vi "CRYEmpty Listbox.vi"   [LabVIEW 2013]
uses:
  Global/CRYCurve Library Global.vi
panel:
  # "Empty Curve Library Listbox"
types:
  T1 = cluster{"Left Cell String":string, "Child Text":string[], "Child Tag":string, "Item Indent":i32, "Child Only?":bool, "Glyph Index":i32}[]
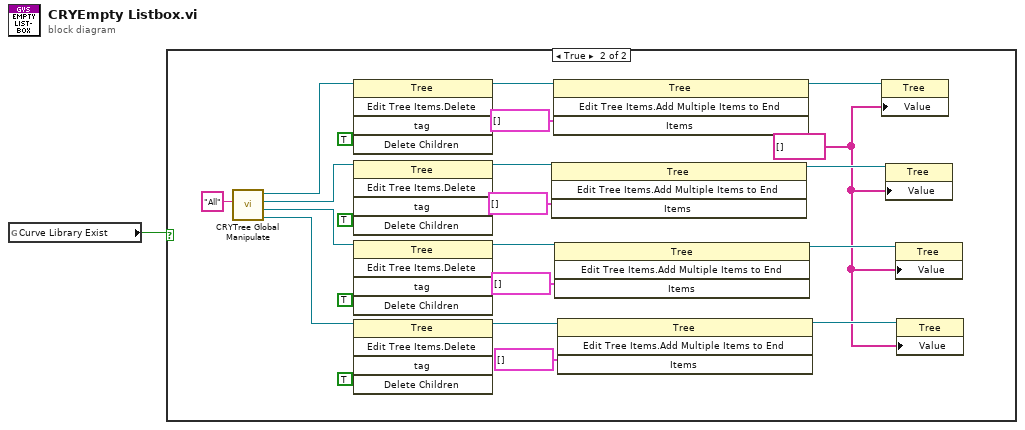
[diagram p0: block diagram]
diagram:
  n1 = global read "CRYCurve Library Global.vi" "Curve Library Exist"() -> (w1:bool)
  n2 = case shown="True" w1 {
    frame False {
    }
    frame True {
      w2 = string[] []
      n3 = call "CRYTree Global Manipulate.vi"("sOption"="All") -> ("WFM Tree"=w10:refnum<vi>, "Results Tree"=w9:refnum<vi>, "Values Tree"=w8:refnum<vi>, "Tree/Curve Tree"=w7:refnum<vi>)  [unwired: 7 in]
      n4 = invoke on="Invoke Node" class="Tree" method="Edit Tree Items.Delete"(reference=w7, "Delete Children"=TRUE ("Delete Children?")) -> (reference out=w19:refnum<vi>)  [unwired: 3 in, 4 out]
      n5 = invoke on="Invoke Node" class="Tree" method="Edit Tree Items.Delete"(reference=w8, "Delete Children"=TRUE ("Delete Children?")) -> (reference out=w13:refnum<vi>)  [unwired: 3 in, 4 out]
      n6 = invoke on="Invoke Node" class="Tree" method="Edit Tree Items.Delete"(reference=w9, "Delete Children"=TRUE ("Delete Children?")) -> (reference out=w14:refnum<vi>)  [unwired: 3 in, 4 out]
      n7 = invoke on="Invoke Node" class="Tree" method="Edit Tree Items.Delete"(reference=w10, "Delete Children"=TRUE ("Delete Children?")) -> (reference out=w12:refnum<vi>)  [unwired: 3 in, 4 out]
      n8 = invoke class="Tree" method="Edit Tree Items.Add Multiple Items to End"(reference=w13, "Items"=T1 []) -> (reference out=w5:refnum<vi>)  [unwired: 2 in, 3 out]
      n9 = invoke class="Tree" method="Edit Tree Items.Add Multiple Items to End"(reference=w19, "Items"=T1 []) -> (reference out=w6:refnum<vi>)  [unwired: 2 in, 3 out]
      n10 = invoke class="Tree" method="Edit Tree Items.Add Multiple Items to End"(reference=w14, "Items"=T1 []) -> (reference out=w4:refnum<vi>)  [unwired: 2 in, 3 out]
      n11 = invoke class="Tree" method="Edit Tree Items.Add Multiple Items to End"(reference=w12, "Items"=T1 []) -> (reference out=w3:refnum<vi>)  [unwired: 2 in, 3 out]
      n12 = property class="Tree"(reference=w6, "Value"=w2) -> ()  [unwired: 1 in, 2 out]
      n13 = property class="Tree"(reference=w5, "Value"=w2) -> ()  [unwired: 1 in, 2 out]
      n14 = property class="Tree"(reference=w4, "Value"=w2) -> ()  [unwired: 1 in, 2 out]
      n15 = property class="Tree"(reference=w3, "Value"=w2) -> ()  [unwired: 1 in, 2 out]
    }
  }
